vi "Get Last Stream.vi"(11 "Data":dbl[][](array[numeric])) -> (3 "Array of Waveform":waveform(dbl)[](array[waveform]))   [LabVIEW 2020]
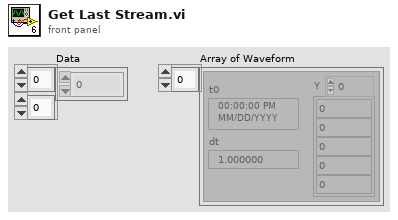
[diagram p1: front panel]
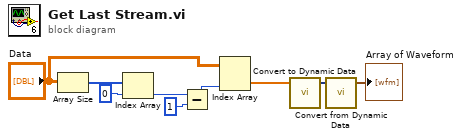
[diagram p0: block diagram]
diagram:
  n1 = Array Size(array="Data") -> (size(s)=w5:i32[])
  n2 = Index Array(array=w5, index=0) -> (element=w3:i32)
  n3 = Subtract(x=w3, y=1) -> (x-y=w1:i32)
  n4 = Index Array(array="Data", index (row)=w1) -> (element=w7:dbl[])  [unwired: 1 in]
  n5 = call "Convert to Dynamic Data"("Array"=w7) -> ("Dynamic Data Type"=w8:dynamicdata)  [unwired: 3 in]
  n6 = call "Convert from Dynamic Data"("Dynamic Data Type"=w8) -> ("Array of Waveform"=→"Array of Waveform":waveform(dbl)[])  [unwired: 3 in]
